vi "Configure.vi"(8 "error in":errorcluster, 9 "Config Handle":T1, 10 "section":string="Serial Config", 11 "Serial Session in":refnum<class "Serial Session.lvclass">) -> (0 "error out":errorcluster, 3 "Serial Session out":refnum<class "Serial Session.lvclass">)   [LabVIEW 2014, in "Serial Session.lvclass"]
doc: "Configure uses an existing configuration file association to configure the port for operation."
uses:
  Serial Session.lvclass
  File Access/Config Data/Config Session.ctl
  File Access/Config Data/Config Data.lvclass
  Typedefs/Serial Config.ctl
  Typedefs/Msg Config.ctl
  File Access/Config Data/Config Data.lvclass/Config Data.ctl
  Serial Session.lvclass/Serial Session.ctl
  File Access/Config Data/Accessors/Read Ref.vi
  <vilib>/Utility/config.llb/Read Key (I32).vi
  <vilib>/Utility/config.llb/Read Key (String).vi
  <vilib>/Utility/config.llb/NI_LVConfig.lvlib
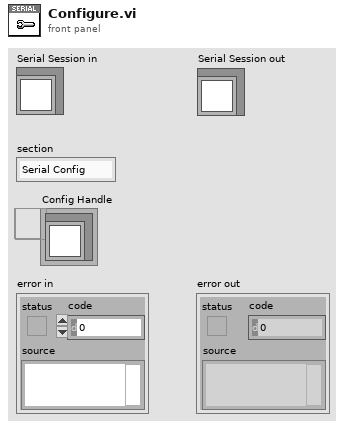
[diagram p1: front panel]
types:
  T1 = typedef "Config Data.lvclass/Config Session.ctl" = refnum<data-value>
  T2 = typedef "Serial Session.lvclass/Msg Config.ctl" = cluster{"sendEndEn":bool, "suppEnEnRd":bool, "termChar":u8, "EnTermChar":bool}
  T3 = typedef "Serial Session.lvclass/Serial Config.ctl" = cluster{"baud rate":u32, "data bits":u16, "stop bits":u16, "parity":u16, "flow control":u16, "endModeforReads":u16, "endModeforWrites":u16}
  T4 = typedef "NI_LVConfig.lvlib/Config Data RefNum.ctl" = refnum<k1>
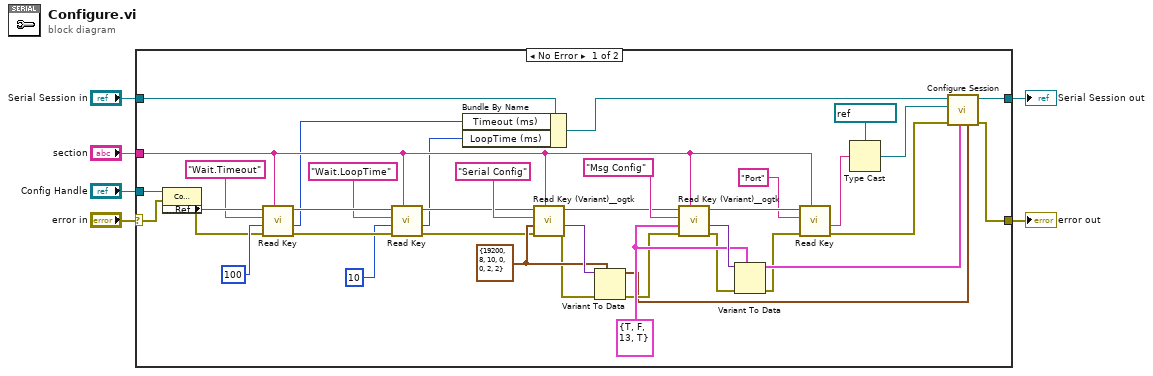
[diagram p0: block diagram]
diagram:
  n1 = case shown="No Error" "error in" {
    selector: "error in" -> [w33 w46]
    tunnel: [w26 w46] -> w5
    tunnel: [w29 w45] -> w3
    tunnel: "Serial Session in" -> [w10 w45]
    tunnel: "Config Handle" -> [w44 _]
    tunnel: "section" -> [w17 _]
    frame No Error {
      w37 = T2 {"sendEndEn"=TRUE, "suppEnEnRd"=FALSE, "termChar"=13, "EnTermChar"=TRUE} ("Msg Configuration")
      w42 = T3 {"baud rate"=19200, "data bits"=8, "stop bits"=10, "parity"=0, "flow control"=0, "endModeforReads"=2, "endModeforWrites"=2} ("Serial Config")
      n2 = property class="Config Data"(reference=w44, error in=w33) -> (error out=w11:errorcluster, "Accessors:Ref"=w21:T4)  [unwired: 1 out]
      n3 = call-poly <vilib>:"Read Key.vi"("section"=w17, "error in (no error)"=w11, "default value"=100, "key"="Wait.Timeout", "refnum"=w21) -> ("error out"=w15:errorcluster, "value"=w9:i32, "refnum out"=w19:T4)  [unwired: 3 in, 1 out]
      n4 = call-poly <vilib>:"Read Key.vi"("section"=w17, "error in (no error)"=w15, "default value"=10, "key"="Wait.LoopTime", "refnum"=w19) -> ("error out"=w12:errorcluster, "value"=w7:i32, "refnum out"=w18:T4)  [unwired: 3 in, 1 out]
      n5 = Bundle By Name(cluster=w10, "Timeout (ms)"=w9, "LoopTime (ms)"=w7) -> (w8:refnum<class "Serial Session.lvclass">)
      n6 = call <userlib>:"Read Key (Variant)__ogtk.vi"("section"=w17, "error in (no error)"=w12, "type"=w42, "key (optional)"="Serial Config", "refnum"=w18) -> ("error out"=w41:errorcluster, "key-value"=w43:variant, "refnum out"=w32:T4)  [unwired: 3 in, 1 out]
      n7 = Variant To Data(error in=w41, type=w42, Variant=w43) -> (data=w25:T3, error out=w36:errorcluster)
      n8 = call <userlib>:"Read Key (Variant)__ogtk.vi"("section"=w17, "error in (no error)"=w36, "type"=w37, "key (optional)"="Msg Config", "refnum"=w32) -> ("error out"=w23:errorcluster, "key-value"=w38:variant, "refnum out"=w35:T4)  [unwired: 3 in, 1 out]
      n9 = Variant To Data(error in=w23, type=w37, Variant=w38) -> (data=w24:T2, error out=w22:errorcluster)
      n10 = call-poly <vilib>:"Read Key.vi"("section"=w17, "error in (no error)"=w22, "key"="Port", "refnum"=w35) -> ("error out"=w28:errorcluster, "value"=w31:string)  [unwired: 4 in, 2 out]
      n11 = Type Cast(type=refnum<visa-resource-name> "COM5" ("VISA Resource"), x=w31) -> (*(type *) &x=w27:refnum<visa-resource-name>)
      n12 = call "Configure Session.vi"("serialCfg"=w25, "Message Cfg"=w24, "error in"=w28, "VISA Resource"=w27, "Serial Session"=w8) -> ("error out"=w26:errorcluster, "Serial Session out"=w29:refnum<class "Serial Session.lvclass">)  [unwired: 5 in]
    }
    frame Error {
    }
  }
  "error out" <- w5
  "Serial Session out" <- w3
